vi "GetFreq.vi"(8 "error in (no error)":errorcluster, 9 "Map":T1, 11 "waveforms":waveform(dbl)[](array[waveform])) -> (0 "error out":errorcluster, 3 "frequency":dbl=60.0)   [LabVIEW 2017, in "McsaAnalysisFunctions.lvlib"]
uses:
  <vilib>/addons/InsightCM/Utilities/Analysis/MCSA/McsaAnalysisFunctions.lvlib
  <vilib>/addons/PointValueMap/controls/PointMap.ctl
  <vilib>/addons/PointValueMap/subVIs/Point_Write_double.vi
  <vilib>/addons/Electrical Power/Basic/NI_EP_Basic.lvlib
  <vilib>/addons/PointValueMap/PointValueMap.lvlib
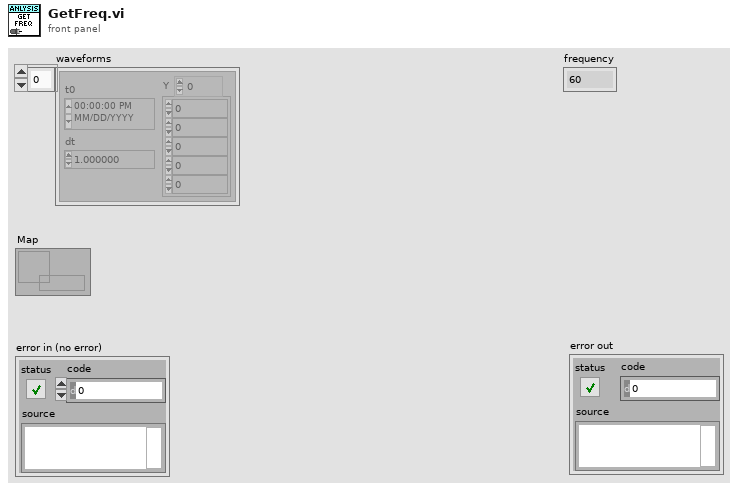
[diagram p1: front panel]
types:
  T1 = typedef "PointValueMap.lvlib/PointMap.ctl" = refnum<data-value>
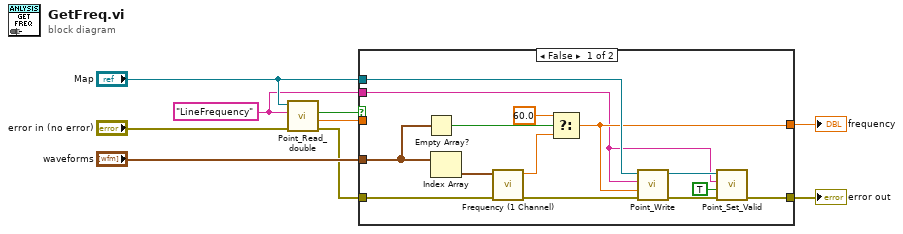
[diagram p0: block diagram]
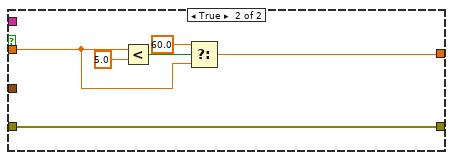
[diagram p2: hidden frame]
diagram:
  w1 = "LineFrequency" ("Tag")
  n1 = call <vilib>:"Point_Read_double.vi"("Error In"="error in (no error)", "Tag"=w1, "Map"="Map") -> ("Error Out"=w4:errorcluster, "Value"=w3:dbl, "Found?"=w6:bool)  [unwired: 3 in, 3 out]
  n2 = case shown="False" w6 {
    tunnel: [w15 w24] -> w7
    tunnel: [w13 w29] -> w8
    tunnel: w4 -> [w23 w29]
    tunnel: "waveforms" -> [w22 _]
    tunnel: w3 -> [_ w25]
    tunnel: "Map" -> [w16 _]
    tunnel: w1 -> [w11 _]
    frame False {
      n3 = Empty Array?(array=w22) -> (empty?=w21:bool)
      n4 = Index Array(array=w22) -> (element=w18:waveform(dbl))  [unwired: 1 in]
      n5 = call <vilib>:"Frequency (1 Channel).vi"("error in (no error)"=w23, "waveform"=w18) -> ("error out"=w17:errorcluster, "frequency"=w20:dbl)  [unwired: 8 in]
      n6 = Select(t=60.0, s=w21, f=w20) -> (s? t:f=w15:dbl)
      n7 = call-poly <vilib>:"Point_Write.vi"("Error In"=w17, "Value"=w15, "Tag"=w11, "Map"=w16) -> ("Error Out"=w14:errorcluster, "Map Out"=w12:T1)  [unwired: 6 in]
      n8 = call <vilib>:"Point_Set_Valid.vi"("Error In"=w14, "Valid?"=TRUE, "Tag"=w11, "Map"=w12) -> ("Error Out"=w13:errorcluster)  [unwired: 6 in, 1 out]
    }
    frame True {
      n9 = Less?(x=w25, y=5.0) -> (x < y?=w27:bool)
      n10 = Select(t=60.0, s=w27, f=w25) -> (s? t:f=w24:dbl)
    }
  }
  "frequency" <- w7
  "error out" <- w8
